vi "Jump.vi"(6 "Single Needle":bool, 8 "Error In":errorcluster, 9 "Strip No.":u16, 10 "Region":u16, 11 "ProbeStationControl in":refnum<class "ProbeStationControl.lvclass">) -> (0 "Error Out":errorcluster, 3 "ProbeStationControl out":refnum<class "ProbeStationControl.lvclass">)   [LabVIEW 2013]
doc: "Move to specified strip index and touch down probe."
uses:
  InstrControl/ProbeStationControl/ProbeStationControl.lvclass
  ProbePlanParams.vi
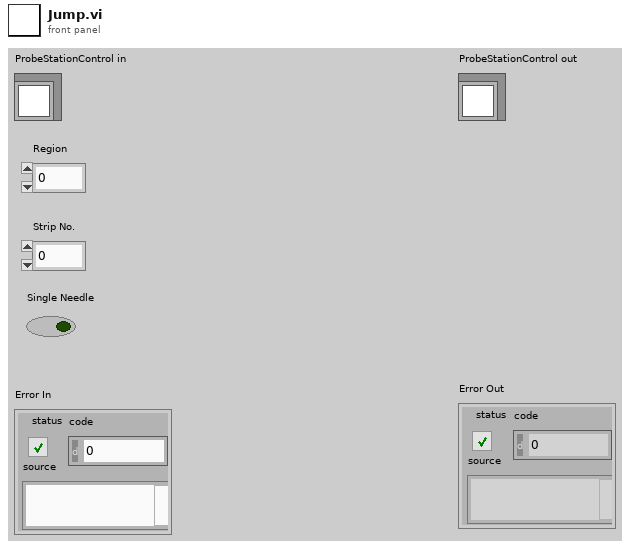
[diagram p1: front panel]
types:
  T1 = cluster{"Strip Number OUT":i32, "X0":i32, "Y0":i32, "X1":i32, "Y1":i32, "Xref":dbl, "Yref":dbl, "ProbePlan type":u32, "Inner pads offset":ext, "Outer pads offset":ext, "l_inner":ext, "l_outer":ext, "strip numbering":u16, "Device Orientation":ext, "Stagger offset":i32, "Yoffset":dbl, "Strip pitch":dbl, "Fiducail separation":dbl, "Radius":ext, "Relative strip angles":dbl, "Probeplan description":string, "ProbePlan array":cluster{"Region":string, "ProbePoints":cluster{"X":dbl, "Y":dbl, "Label":string, "CardViable?":bool}[]}[], "Test ProbePoints":cluster{"Regions Enabled":bool[], "From index":u32[], "To index":u32[], "Strip length [cm]":dbl[]}}
  T2 = cluster{"Region":string, "ProbePoints":cluster{"X":dbl, "Y":dbl, "Label":string, "CardViable?":bool}[]}[]
  T3 = cluster{"Region":string, "ProbePoints":cluster{"X":dbl, "Y":dbl, "Label":string, "CardViable?":bool}[]}
  T4 = cluster{"X":dbl, "Y":dbl, "Label":string, "CardViable?":bool}[]
  T5 = cluster{"X":dbl, "Y":dbl, "Label":string, "CardViable?":bool}
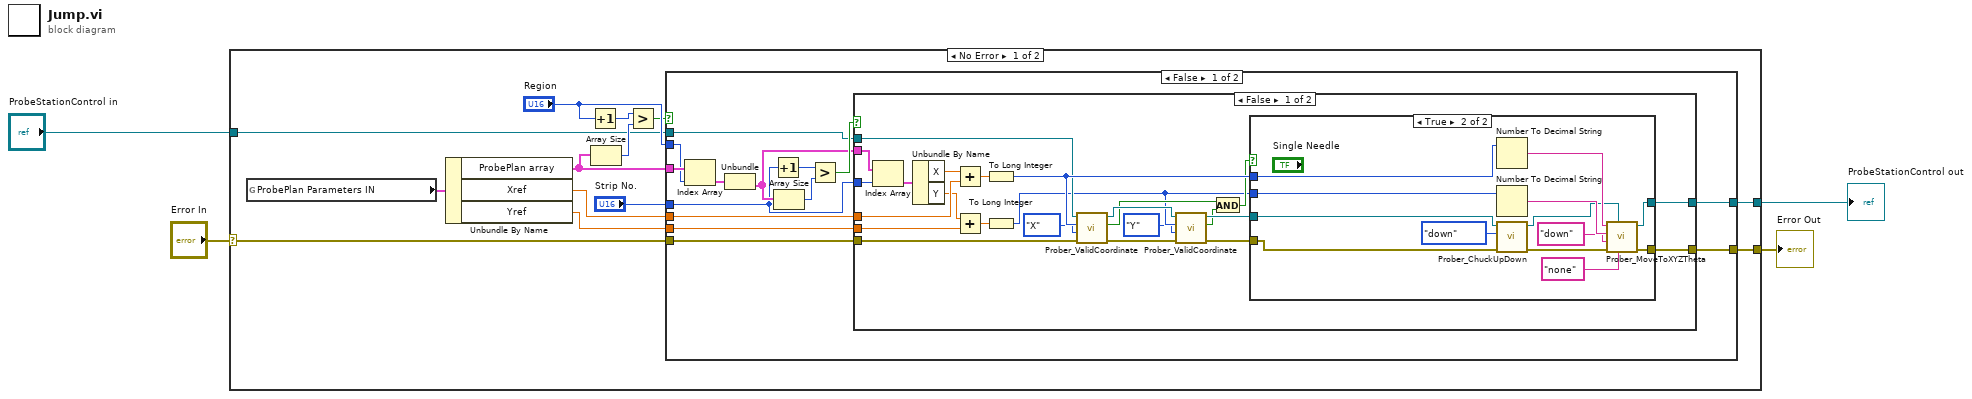
[diagram p0: block diagram]
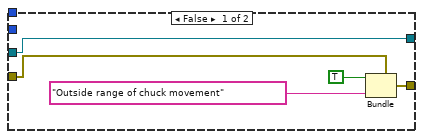
[diagram p2: hidden frame]
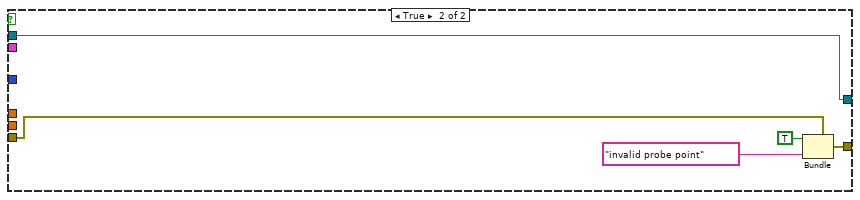
[diagram p3: hidden frame]
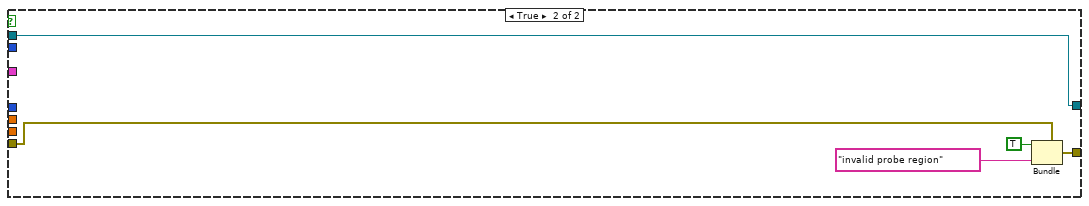
[diagram p4: hidden frame]
diagram:
  n1 = case shown="No Error" "Error In" {
    selector: "Error In" -> [w11 w84]
    tunnel: [w17 w84] -> w4
    tunnel: "ProbeStationControl in" -> [w5 w85]
    tunnel: [w6 w85] -> w1
    frame No Error {
      n2 = global read "ProbePlanParams.vi" "ProbePlan Parameters IN"() -> (w10:T1)
      n3 = Unbundle By Name(w10) -> ("ProbePlan array"=w9:T2, "Xref"=w8:dbl, "Yref"=w7:dbl)
      n4 = Increment(x="Region") -> (x+1=w13:u16)
      n5 = Array Size(array=w9) -> (size(s)=w14:i32)
      n6 = Greater?(x=w13, y=w14) -> (0:w12:bool)
      n7 = case shown="False" w12 {
        tunnel: w11 -> [w26 w83]
        tunnel: [w25 w82] -> w17
        tunnel: "Region" -> [w29 _]
        tunnel: "Strip No." -> [w20 _]
        tunnel: w9 -> [w30 _]
        tunnel: w7 -> [w23 _]
        tunnel: w8 -> [w22 _]
        tunnel: [w19 w79] -> w6
        tunnel: w5 -> [w18 w79]
        frame False {
          n8 = Index Array(array=w30, index=w29) -> (element=w31:T3)
          n9 = Unbundle(w31) -> ("ProbePoints"=w21:T4)  [unwired: 1 out]
          n10 = Increment(x=w20) -> (x+1=w27:u16)
          n11 = Array Size(array=w21) -> (size(s)=w28:i32)
          n12 = Greater?(x=w27, y=w28) -> (0:w24:bool)
          n13 = case shown="False" w24 {
            tunnel: w26 -> [w42 w77]
            tunnel: [w48 w76] -> w25
            tunnel: w23 -> [w55 _]
            tunnel: w22 -> [w54 _]
            tunnel: w21 -> [w53 _]
            tunnel: w20 -> [w52 _]
            tunnel: [w45 w74] -> w19
            tunnel: w18 -> [w43 w74]
            frame False {
              n14 = Index Array(array=w53, index=w52) -> (element=w51:T5)
              n15 = Unbundle By Name(w51) -> ("X"=w50:dbl, "Y"=w49:dbl)
              n16 = Add(x=w50, y=w54) -> (x+y=w47:dbl)
              n17 = Add(x=w49, y=w55) -> (x+y=w46:dbl)
              n18 = To Long Integer(number=w47) -> (32bit integer=w44:i32)
              n19 = To Long Integer(number=w46) -> (32bit integer=w34:i32)
              n20 = call-dynamic "Prober_ValidCoordinate.vi"("error in (no error)"=w42, "Axis"=enum16{"X", "Y", "Z", "Theta"}."X", "Coordinate IN"=w44, "ProbeStationControl in"=w43) -> ("error out"=w41:errorcluster, "Is Valid?"=w36:bool, "ProbeStationControl out"=w39:refnum<class "ProbeStationControl.lvclass">)  [unwired: 5 in]
              n21 = call-dynamic "Prober_ValidCoordinate.vi"("error in (no error)"=w41, "Axis"=enum16{"X", "Y", "Z", "Theta"}."Y", "Coordinate IN"=w34, "ProbeStationControl in"=w39) -> ("error out"=w40:errorcluster, "Is Valid?"=w37:bool, "ProbeStationControl out"=w38:refnum<class "ProbeStationControl.lvclass">)  [unwired: 5 in]
              n22 = And(x=w36, y=w37) -> (x .and. y?=w35:bool)
              n23 = case shown="True" w35 {
                tunnel: w40 -> [w58 w63]
                tunnel: [w57 w62] -> w48
                tunnel: w44 -> [_ w73]
                tunnel: w34 -> [_ w72]
                tunnel: [w56 w61] -> w45
                tunnel: w38 -> [w56 w64]
                frame False {
                  n24 = Bundle(cluster=w58, "status"=TRUE, "source"="Outside range of chuck movement") -> (w57:errorcluster)  [unwired: 1 in]
                }
                frame True {
                  n25 = Number To Decimal String(number=w73) -> (decimal integer string=w71:string)  [unwired: 1 in]
                  n26 = Number To Decimal String(number=w72) -> (decimal integer string=w70:string)  [unwired: 1 in]
                  n27 = call-dynamic "Prober_ChuckUpDown.vi"("error in (no error)"=w63, "Direction"=enum16{"up", "down"}."down", "ProbeStationControl in"=w64) -> ("error out"=w66:errorcluster, "ProbeStationControl out"=w67:refnum<class "ProbeStationControl.lvclass">)  [unwired: 6 in, 1 out]
                  n28 = call-dynamic "Prober_MoveToXYZTheta.vi"("Theta location [mdeg]"="none", "ProbeStationControl in"=w67, "error in (no error)"=w66, "Z location [µm]"="down", "Y location [µm]"=w70, "X location [µm]"=w71) -> ("error out"=w62:errorcluster, "ProbeStationControl out"=w61:refnum<class "ProbeStationControl.lvclass">)  [unwired: 3 in, 1 out]
                }
              }
            }
            frame True {
              n29 = Bundle(cluster=w77, "status"=TRUE, "source"="invalid probe point") -> (w76:errorcluster)  [unwired: 1 in]
            }
          }
        }
        frame True {
          n30 = Bundle(cluster=w83, "status"=TRUE, "source"="invalid probe region") -> (w82:errorcluster)  [unwired: 1 in]
        }
      }
    }
    frame Error {
    }
  }
  "Error Out" <- w4
  "ProbeStationControl out" <- w1
